vi "Test1_2bis.vi"(0 "Instrument VISA in":T1={"AWG VISA"="81160A", "Oscilloscope  VISA "="DSO80204B", "Integration Board IP"="172.16.7.43", "connection ID"=refnum, "report out"=refnum}, 2 "Report Enable":bool, 5 "DT_50_L0":i32[][](array[numeric]), 7 "Cycles Burst":i32=10000, 11 "error in":errorcluster) -> (4 "Instrument VISA out":T1={"AWG VISA"="81160A", "Oscilloscope  VISA "="DSO80204B", "Integration Board IP"="172.16.7.43", "connection ID"=refnum, "report out"=refnum}, 15 "error out":errorcluster)   [LabVIEW 2009]
doc: "This VI provides the distribution of the detected IPR using different pulse amplitudes."
uses:
  <instrlib>/Agilent 81150/Agilent 81150.lvlib
  <vilib>/gmath/NI_Gmath.lvlib
  <vilib>/Utility/NIReport.llb/NI_report.lvclass
  <vilib>/Utility/NIReport.llb/Append Report Text (str wrap).vi
  <vilib>/Utility/NIReport.llb/Append Text Table to Report (wrap).vi
  <vilib>/express/express signal manip/GetorSetDDTAttributes/Shared VIs/XDimension.ctl
  <vilib>/express/express signal manip/GetorSetDDTAttributes/Shared VIs/GetSetShared.lvlib
  <vilib>/express/express signal manip/GetorSetDDTAttributes/Set DDT Attributes/Set DDT Properties.xnode
  <vilib>/express/express shared/transition.llb/Dynamic To Waveform Array.vi
  <vilib>/express/express signal manip/GetorSetDDTAttributes/Shared VIs/XDimension Enum to String.vi
  <vilib>/express/express signal manip/GetorSetDDTAttributes/Set DDT Attributes/SetT0.vi
  <vilib>/express/express shared/transition.llb/Waveform Array To Dynamic.vi
panel:
  out "IPR value":i32
  in  "Curve data path":path=path "D:/CTA/IntegrationBoard/tmp"
  in  "Save curves":bool
  out "XY Graph 2":cluster{"Y":dbl[], "Y":dbl[]}[](graph)
  out "XY Graph":cluster{"Y":dbl[], "Y":dbl[]}[](graph)
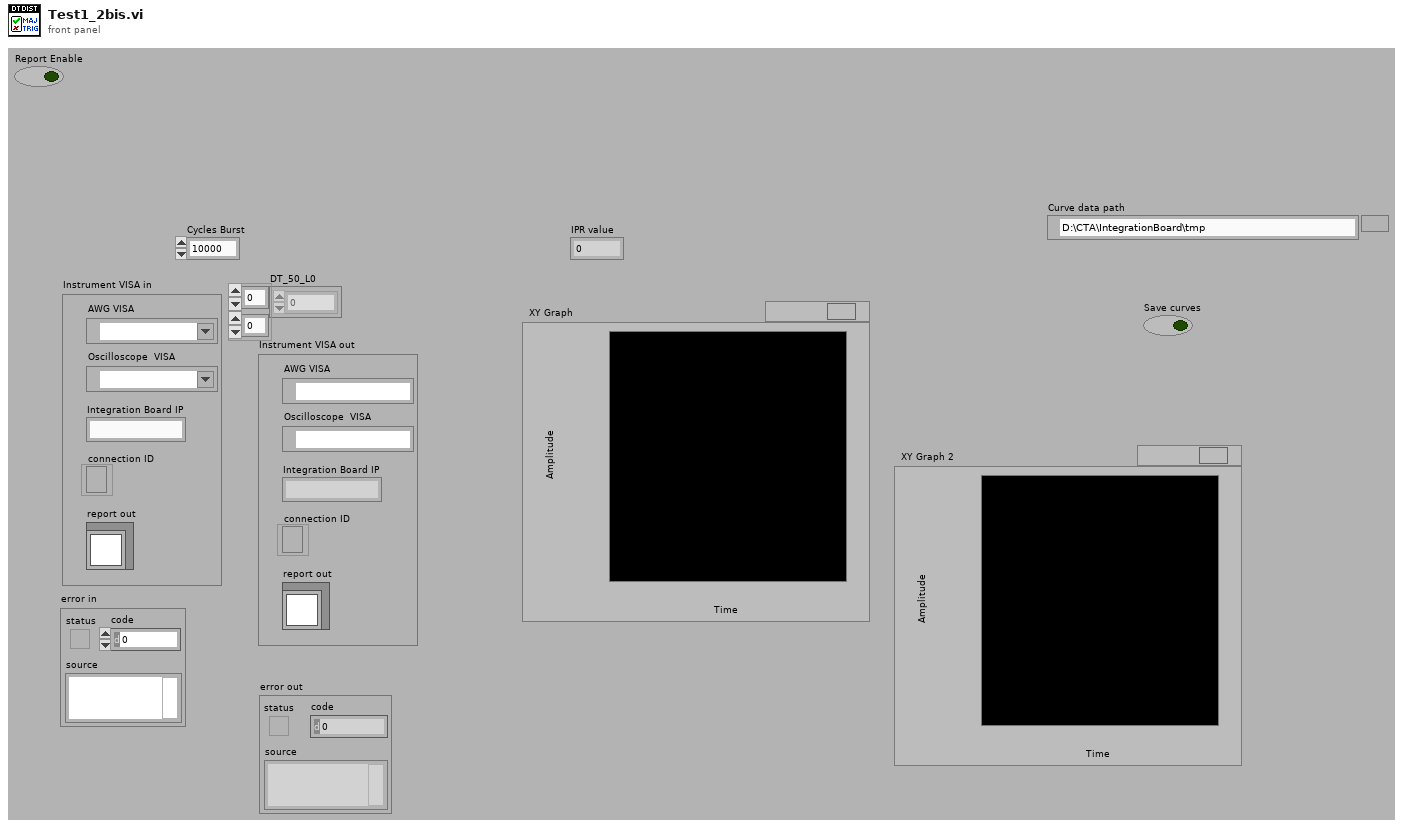
[diagram p1: front panel]
types:
  T1 = cluster{"AWG VISA":refnum<visa-resource-name>, "Oscilloscope  VISA ":refnum<visa-resource-name>, "Integration Board IP":string, "connection ID":refnum<k5>, "report out":refnum<class "NI_report.lvclass">}
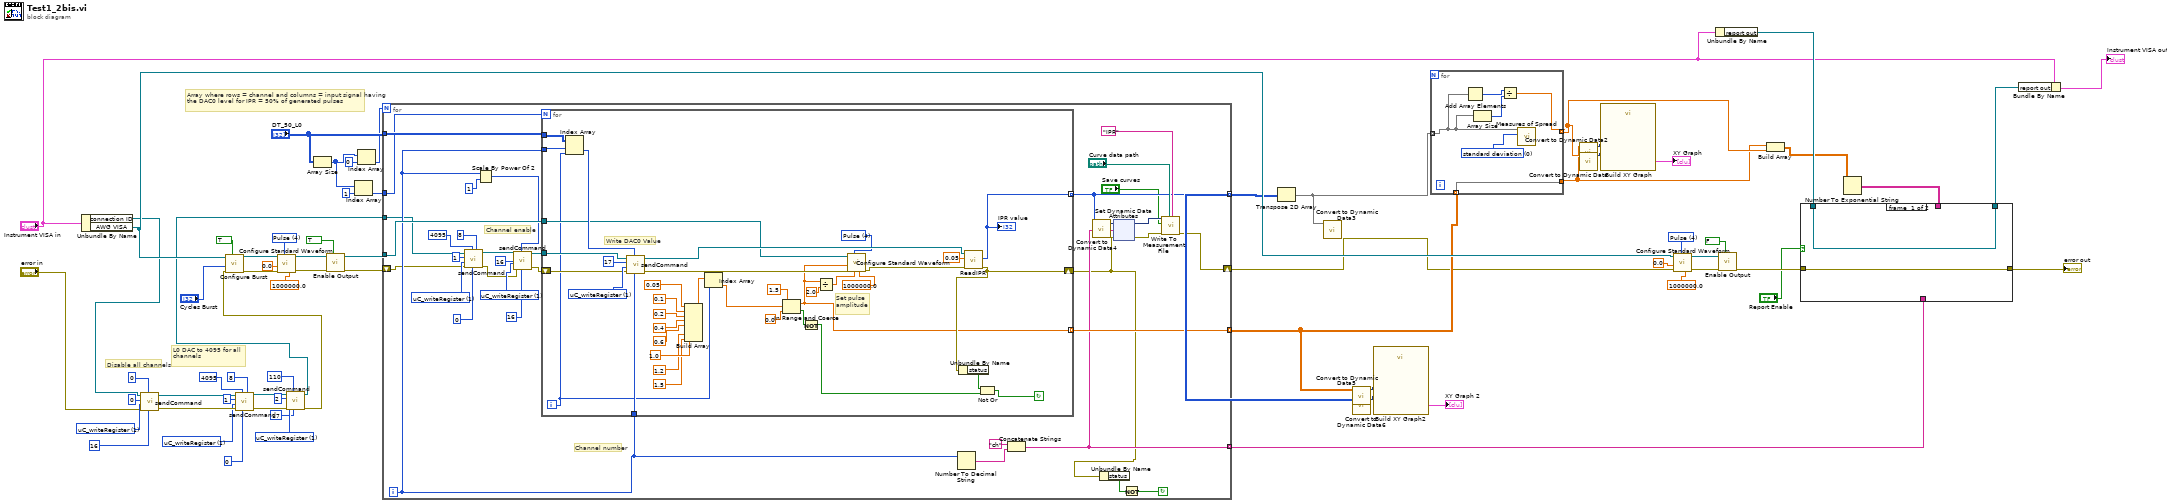
[diagram p0: block diagram]
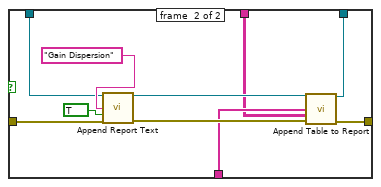
[diagram p2: hidden frame]
diagram:
  w17 = u16 1 items=["sendCommand"=9, "FPGA_writeRegister"=3, "FPGA_readRegister"=2, "uC_writeRegister"=1, "uC_readRegister"=0] ("Action")
  w31 = u16 1 items=["sendCommand"=9, "FPGA_writeRegister"=3, "FPGA_readRegister"=2, "uC_writeRegister"=1, "uC_readRegister"=0] ("Action")
  w37 = u16 1 items=["sendCommand"=9, "FPGA_writeRegister"=3, "FPGA_readRegister"=2, "uC_writeRegister"=1, "uC_readRegister"=0] ("Action")
  w55 = u16 4 items=["Sine", "Square", "Ramp Up", "Ramp Down", "Pulse", "Noise", "DC"] ("Waveform (0: Sine)")
  w67 = u16 4 items=["Sine", "Square", "Ramp Up", "Ramp Down", "Pulse", "Noise", "DC"] ("Waveform (0: Sine)")
  # "Disable all channels"
  # "L0 DAC to 4095 for all channels"
  # "Array where rows = channel and columns = input signal having the DAC0 level for IPR = 50% of generated pulses"
  n1 = Unbundle By Name("Instrument VISA in") -> ("connection ID"=w25:refnum<k5>, "AWG VISA"=w50:refnum<visa-resource-name>)
  n2 = call "sendCommand.vi"("Address"=16, "Data"=0, "error in"="error in", "Action"=w37, "id_in"=0 ("id"), "connection ID"=w25) -> ("error out"=w33:errorcluster, "connection ID out"=w32:refnum<k5>)  [unwired: 1 in, 3 out]
  n3 = call "sendCommand.vi"("number data"=8, "Address"=0, "Data"=4095, "error in"=w33, "Action"=w31, "id_in"=1 ("id"), "connection ID"=w32) -> ("error out"=w22:errorcluster, "connection ID out"=w20:refnum<k5>)  [unwired: 3 out]
  n4 = call "sendCommand.vi"("Address"=17, "Data"=110, "error in"=w22, "Action"=w17, "id_in"=2 ("id"), "connection ID"=w20) -> ("error out"=w23:errorcluster, "connection ID out"=w21:refnum<k5>)  [unwired: 1 in, 3 out]
  n5 = call <instrlib>:"Configure Burst.vi"("Enable Burst (F: Disable)"=TRUE, "error in (no error)"=w23, "Burst Count (2)"="Cycles Burst", "VISA resource name"=w50) -> ("error out"=w64:errorcluster, "VISA resource name out"=w65:refnum<visa-resource-name>)  [unwired: 6 in]
  n6 = call <instrlib>:"Configure Standard Waveform.vi"("Frequency (1000.0 Hz)"=1000000.0, "Waveform (0: Sine)"=w67, "error in (no error)"=w64, "Amplitude (1.0 Vpp)"=0.0, "VISA resource name"=w65) -> ("error out"=w63:errorcluster, "VISA resource name out"=w62:refnum<visa-resource-name>)  [unwired: 5 in]
  n7 = Array Size(array="DT_50_L0") -> (size(s)=w40:i32[])
  n8 = call <instrlib>:"Enable Output.vi"("Enable Output (T: Enable)"=TRUE, "error in (no error)"=w63, "VISA resource name"=w62) -> ("error out"=w58:errorcluster, "VISA resource name out"=w57:refnum<visa-resource-name>)  [unwired: 7 in]
  n9 = Index Array(array=w40, index=1) -> (element=w38:i32)
  n10 = Index Array(array=w40, index=0) -> (element=w24:i32)
  n11 = for {
    N: w24 -> [_]
    shift-right: [w69] -> w6
    shift-left: w58 -> [w88]
    tunnel: w57 -> [w98]
    tunnel: w21 -> [w87]
    tunnel: "DT_50_L0" -> [w97]
    tunnel: [w71] -> w9 mode=indexing
    tunnel: w38 -> [w84]
    tunnel: [w74] -> w7 mode=indexing
    tunnel: [w79] -> w8 mode=indexing
    i -> [w94]
    stop <- w81 continue-if-true
    w93 = u16 1 items=["sendCommand"=9, "FPGA_writeRegister"=3, "FPGA_readRegister"=2, "uC_writeRegister"=1, "uC_readRegister"=0] ("Action")
    w103 = u16 1 items=["sendCommand"=9, "FPGA_writeRegister"=3, "FPGA_readRegister"=2, "uC_writeRegister"=1, "uC_readRegister"=0] ("Action")
    # "Channel number"
    # "Channel enable"
    n12 = call "sendCommand.vi"("number data"=8, "Address"=0, "Data"=4095, "error in"=w88, "Action"=w93, "id_in"=1 ("id"), "connection ID"=w87) -> ("error out"=w85:errorcluster, "connection ID out"=w86:refnum<k5>)  [unwired: 3 out]
    n13 = Scale By Power Of 2(n=w94, x=1) -> (x*2^n=w82:i32)
    n14 = call "sendCommand.vi"("Address"=16 ("Data"), "Data"=w82, "error in"=w85, "Action"=w103, "id_in"=16 ("id"), "connection ID"=w86) -> ("error out"=w100:errorcluster, "connection ID out"=w99:refnum<k5>)  [unwired: 1 in, 3 out]
    n15 = for {
      N: w84 -> [_]
      shift-right: [w127] -> w70
      shift-left: w100 -> [w155]
      tunnel: w99 -> [w151]
      tunnel: w98 -> [w149]
      tunnel: w97 -> [w156]
      tunnel: w94 -> [w157]
      tunnel: w94 -> [w154]
      tunnel: [w125] -> w74 mode=indexing
      tunnel: [w123] -> w79 mode=indexing
      i -> [w130]
      stop <- w126 continue-if-true
      w145 = u16 4 items=["Sine", "Square", "Ramp Up", "Ramp Down", "Pulse", "Noise", "DC"] ("Waveform (0: Sine)")
      w159 = u16 1 items=["sendCommand"=9, "FPGA_writeRegister"=3, "FPGA_readRegister"=2, "uC_writeRegister"=1, "uC_readRegister"=0] ("Action")
      # "Set pulse amplitude"
      # "Write DAC0 Value"
      n16 = Index Array(array=w156, index (row)=w157, index (col)=w130) -> (element=w153:i32)
      n17 = call "sendCommand.vi"("Address"=w154, "Data"=w153, "error in"=w155, "Action"=w159, "id_in"=17 ("id"), "connection ID"=w151) -> ("error out"=w152:errorcluster, "connection ID out"=w150:refnum<k5>)  [unwired: 1 in, 3 out]
      n18 = Build Array(0.05 ("element"), 0.1 ("element"), 0.2 ("element"), 0.4 ("element"), 0.6 ("element"), 1.0 ("element"), 1.2 ("element"), 1.5 ("element")) -> (w124:dbl[])
      n19 = Index Array(array=w124, index=w130) -> (element=w128:dbl)
      n20 = In Range and Coerce(upper limit=1.5, x=w128, lower limit=0.0) -> (coerced(x)=w123:dbl, In Range?=w148:bool)
      n21 = Not(x=w148) -> (.not. x?=w142:bool)
      n22 = Divide(x=w123, y=2.0) -> (x/y=w139:dbl)
      n23 = call <instrlib>:"Configure Standard Waveform.vi"("Frequency (1000.0 Hz)"=1000000.0, "DC Offset (0.0 Volts)"=w139, "Waveform (0: Sine)"=w145, "error in (no error)"=w152, "Amplitude (1.0 Vpp)"=w123, "VISA resource name"=w149) -> ("error out"=w138:errorcluster)  [unwired: 4 in, 1 out]
      n24 = call "ReadIPR.vi"("error in"=w138, 10:0.05 ("Delay Time (s)"), "connection ID"=w150) -> ("error out"=w127:errorcluster, "IPR value"=w125:i32)  [unwired: 6 in, 1 out]
      "IPR value" <- w125
      n25 = Unbundle By Name(w127) -> ("status"=w143:bool)
      n26 = Not Or(1:w142, 2:w143) -> (0:w126:bool)
    }
    n27 = Number To Decimal String(number=w94) -> (decimal integer string=w95:string)  [unwired: 1 in]
    n28 = Concatenate Strings("ch" ("string"), w95) -> (w71:string)
    n29 = call "Convert to Dynamic Data4"("Array"=w74) -> ("Dynamic Data Type"=w73:dynamicdata)  [unwired: 3 in]
    n30 = Unbundle By Name(w70) -> ("status"=w80:bool)
    n31 = xnode ("Set Dynamic Data Attributes")("Signals In"=w73, "error in"=w70, "Signal Name"=w71) -> ("Signals Out"=w77:dynamicdata, "error out"=w78:errorcluster)  [unwired: 2 in]
    n32 = Not(x=w80) -> (.not. x?=w81:bool)
    n33 = call "Write To Measurement File"("Signals"=w77, "Enable"="Save curves", "error in (no error)"=w78, "Filename"="Curve data path", "Comment"="IPR" ("Y Signal Name")) -> ("error out"=w69:errorcluster)  [unwired: 12 in, 2 out]
  }
  n34 = Transpose 2D Array(2D array=w7) -> (transposed array=w11:i32[][])
  n35 = call "Convert to Dynamic Data3"("2D Array"=w11) -> ()  [unwired: 3 in, 1 out]
  n36 = call "Convert to Dynamic Data5"("2D Array"=w8) -> ("Dynamic Data Type"=w12:dynamicdata)  [unwired: 3 in]
  n37 = call "Convert to Dynamic Data6"("2D Array"=w7) -> ("Dynamic Data Type"=w10:dynamicdata)  [unwired: 3 in]
  n38 = call "Build XY Graph2"("Y Input"=w10, "X Input"=w12) -> ("XY Graph"=→"XY Graph 2":cluster{"Y":dbl[], "Y":dbl[]}[])  [unwired: 8 in, 1 out]
  n39 = for {
    tunnel: w11 -> [w163] mode=indexing
    tunnel: [w160] -> w2 mode=indexing
    tunnel: w8 -> [w164] mode=indexing
    tunnel: [w164] -> w1
    w165 = 0 items=["standard deviation", "range", "mean absolute deviation", "interquartile range"] ("type")
    n40 = Add Array Elements(numeric array=w163) -> (sum=w162:i32)
    n41 = Array Size(array=w163) -> (size(s)=w161:i32)
    n42 = Divide(x=w162, y=w161) -> (x/y=w160:dbl)
    n43 = call <vilib>:"Measures of Spread.vi"("type"=w165, "x array"=w163) -> ()  [unwired: 8 in, 2 out]
  }
  n44 = call "Convert to Dynamic Data2"("Array"=w1) -> ("Dynamic Data Type"=w14:dynamicdata)  [unwired: 3 in]
  n45 = call "Convert to Dynamic Data"("Array"=w2) -> ("Dynamic Data Type"=w15:dynamicdata)  [unwired: 3 in]
  n46 = call "Build XY Graph"("Y Input"=w15, "X Input"=w14) -> ("XY Graph"=→"XY Graph":cluster{"Y":dbl[], "Y":dbl[]}[])  [unwired: 8 in, 1 out]
  n47 = call <instrlib>:"Configure Standard Waveform.vi"("Frequency (1000.0 Hz)"=1000000.0, "Waveform (0: Sine)"=w55, "error in (no error)"=w6, "Amplitude (1.0 Vpp)"=0.0, "VISA resource name"=w50) -> ("error out"=w52:errorcluster, "VISA resource name out"=w51:refnum<visa-resource-name>)  [unwired: 5 in]
  n48 = Unbundle By Name("Instrument VISA in") -> ("report out"=w49:refnum<class "NI_report.lvclass">)
  n49 = call <instrlib>:"Enable Output.vi"("Enable Output (T: Enable)"=FALSE, "error in (no error)"=w52, "VISA resource name"=w51) -> ("error out"=w48:errorcluster)  [unwired: 7 in, 1 out]
  n50 = Build Array(w1, w2) -> (w4:dbl[][])
  n51 = Number To Exponential String(number=w4) -> (E-format string=w3:string[][])  [unwired: 3 in]
  n52 = case shown="True" "Report Enable" {
    tunnel: [w166 w177] -> w47
    tunnel: w48 -> [w166 w176]
    tunnel: w49 -> [w167 w171]
    tunnel: [w167 w170] -> w43
    tunnel: w9 -> [_ w169]
    tunnel: w3 -> [_ w168]
    frame #0 {
    }
    frame #1 {
      n53 = call-poly <vilib>:"Append Report Text.vi"("report in"=w171, "text"="Gain Dispersion", "append on new line? (F)"=TRUE, "error in (no error)"=w176) -> ("report out"=w172:refnum<class "NI_report.lvclass">, "error out"=w175:errorcluster)  [unwired: 8 in, 2 out]
      n54 = call-poly <vilib>:"Append Table to Report.vi"("report in"=w172, "row headers"=w169, "text data"=w168, "error in (no error)"=w175) -> ("report out"=w170:refnum<class "NI_report.lvclass">, "error out"=w177:errorcluster)  [unwired: 8 in, 2 out]
    }
  }
  "error out" <- w47
  n55 = Bundle By Name(cluster="Instrument VISA in", "report out"=w43) -> (→"Instrument VISA out":T1)
